vi "SiosIfmAirPressure.vi"(1 "Channel":i32(knob) scale=1.0..4.0, 2 "Device Number":i32) -> (0 "Air Pressure":dbl)   [LabVIEW 2009]
uses:
  siosifm.dll
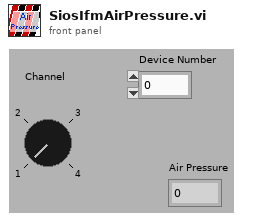
[diagram p1: front panel]
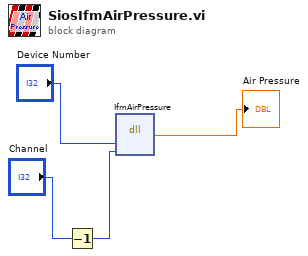
[diagram p0: block diagram]
diagram:
  n1 = Decrement(x="Channel") -> (x-1=w1:i32)
  n2 = dll-call lib="C:/WORK/Artem/RE-10/SIOS_IfmDLL/siosifm.dll" fn="IfmAirPressure"("devNumber"="Device Number", "channel"=w1) -> ("air_pressure"=→"Air Pressure":dbl)  [unwired: 5 in, 2 out]
